vi "Tutorial_7_secondTry.vi"() -> ()   [LabVIEW 2020]
uses:
  <vilib>/Utility/file.llb/Write Delimited Spreadsheet (string).vi
panel:
  out "bytes written 2":i32
  out "bytes written":i32
  out "data out":string
  out "error out":errorcluster
  in  "file path (dialog if empty)":path
  in  "Tab Control":enum32{"Page 1", "Page 2"}(tab)
  in  "Register":bool
  in  "tbl Registration":string[][](table)
  in  "Login UI":enum32{"Page 1", "Page 2"}(tab)
  out "Status":bool
  in  "LoginBtn":bool
  in  "Password":string
  in  "User Name":string
  # "Client"
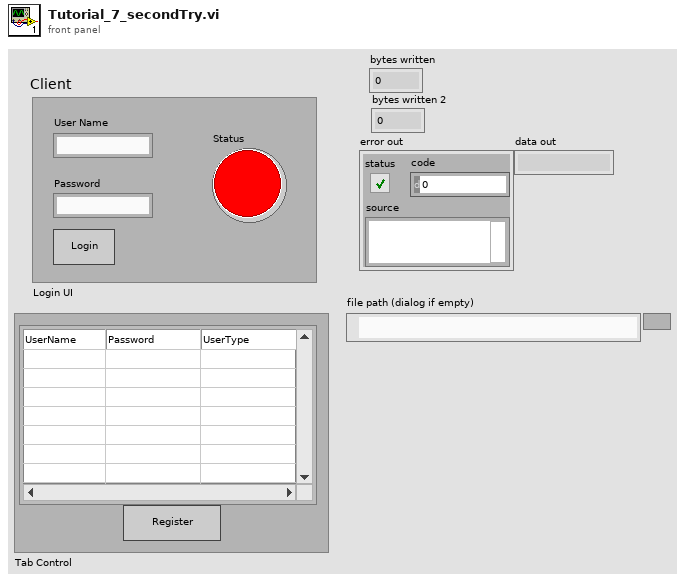
[diagram p1: front panel]
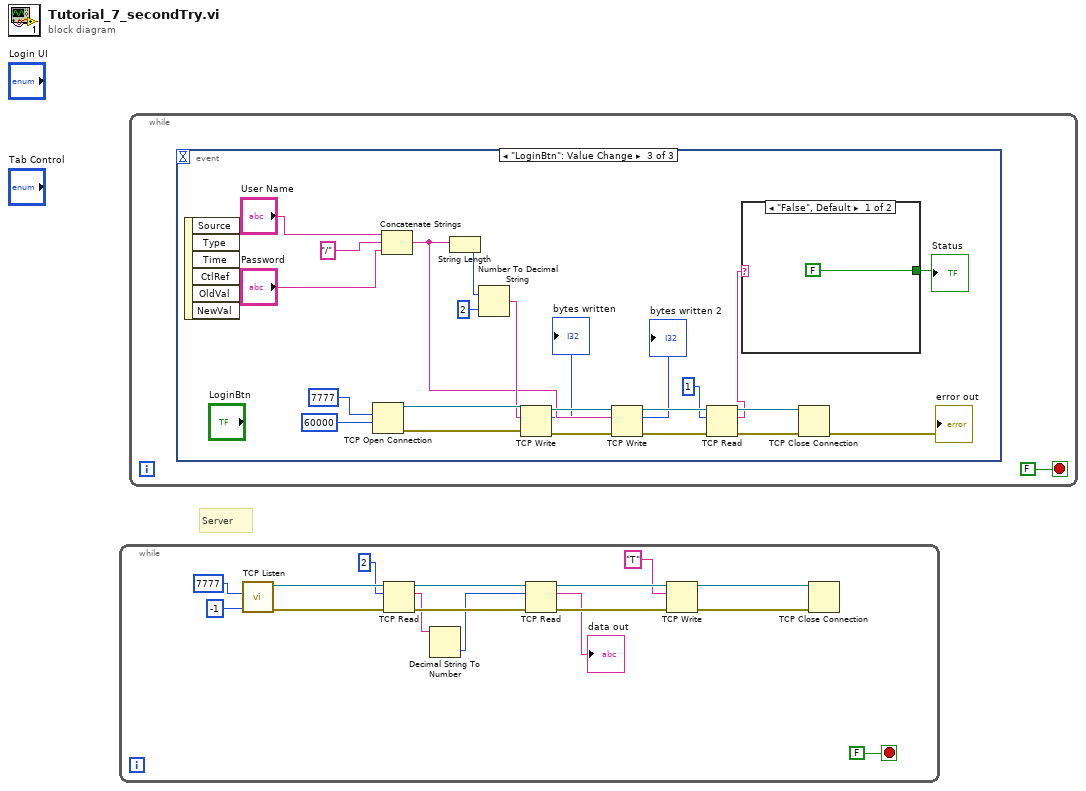
[diagram p0: block diagram]
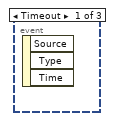
[diagram p2: hidden frame]
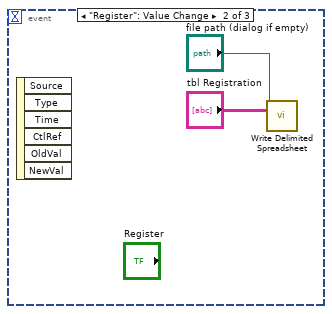
[diagram p3: hidden frame]
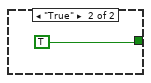
[diagram p4: hidden frame]
diagram:
  # "Server"
  n1 = while {
    stop <- FALSE stop-if-true
    n2 = call <vilib>:"TCP Listen.vi"("timeout ms (wait forever: -1)"=-1, "port"=u16 7777) -> ("error out"=w15:errorcluster, "connection ID"=w16:refnum<k5>)  [unwired: 5 in, 3 out]
    n3 = TCP Read(connection ID=w16, bytes to read=2, error in (no error)=w15) -> (connection ID out=w9:refnum<k5>, data out=w2:string, error out=w14:errorcluster)  [unwired: 2 in]
    n4 = Decimal String To Number(string=w2) -> (number=w3:i32)  [unwired: 2 in, 1 out]
    n5 = TCP Read(connection ID=w9, bytes to read=w3, error in (no error)=w14) -> (connection ID out=w10:refnum<k5>, data out=→"data out":string, error out=w13:errorcluster)  [unwired: 2 in]
    n6 = TCP Write(connection ID=w10, data in="T", error in (no error)=w13) -> (connection ID out=w11:refnum<k5>, error out=w12:errorcluster)  [unwired: 1 in, 1 out]
    n7 = TCP Close Connection(connection ID=w11, error in (no error)=w12) -> ()  [unwired: 1 in, 2 out]
  }
  n8 = while {
    stop <- FALSE stop-if-true
    n9 = event shown="[2] \"LoginBtn\": Value Change" {
      selector: _ -> [_ _ _]
      dyn-events: _ -> [_ _ _]
      timeout: _ -> [_ _ _]
      event Timeout {
        n10 = event-data() -> ()  [unwired: 1 in, 3 out]
      }
      event "Register": Value Change {
        n11 = event-data() -> ()  [unwired: 1 in, 6 out]
        n12 = call-poly <vilib>:"Write Delimited Spreadsheet.vi"("file path (dialog if empty)"="file path (dialog if empty)", "2D data"="tbl Registration") -> ()  [unwired: 12 in, 2 out]
      }
      event "LoginBtn": Value Change {
        n13 = event-data() -> ()  [unwired: 1 in, 6 out]
        n14 = TCP Open Connection(remote port or service name=u16 7777, timeout ms (60000)=60000) -> (connection ID=w38:refnum<k5>, error out=w40:errorcluster)  [unwired: 3 in]
        n15 = Concatenate Strings "Concatenate Strings"("User Name", "/" ("string"), "Password") -> (w27:string)
        n16 = String Length(string=w27) -> (length=w34:i32)
        n17 = Number To Decimal String(number=w34, width (-)=i16 2) -> (decimal integer string=w28:string)
        n18 = TCP Write(connection ID=w38, data in=w28, error in (no error)=w40) -> (connection ID out=w32:refnum<k5>, bytes written=→"bytes written":i32, error out=w29:errorcluster)  [unwired: 1 in]
        n19 = TCP Write(connection ID=w32, data in=w27, error in (no error)=w29) -> (connection ID out=w31:refnum<k5>, bytes written=→"bytes written 2":i32, error out=w30:errorcluster)  [unwired: 1 in]
        n20 = TCP Read(connection ID=w31, bytes to read=1, error in (no error)=w30) -> (connection ID out=w41:refnum<k5>, data out=w25:string, error out=w42:errorcluster)  [unwired: 2 in]
        n21 = case shown="\"False\", Default" w25 {
          tunnel: [FALSE TRUE] -> w24
          frame "False", Default {
          }
          frame "True" {
          }
        }
        "Status" <- w24
        n22 = TCP Close Connection(connection ID=w41, error in (no error)=w42) -> (error out=→"error out":errorcluster)  [unwired: 1 in, 1 out]
      }
    }
  }
